vi "探头校准标准值显示.vi"(11 "校准参数":u16(ring) caption="校准参数：" items=["pH", "DO", "浊度", "电导率", "叶绿素a", "藻密度", "ORP", "DO2"]) -> (1 "标液三":sgl, 2 "标液二":sgl, 3 "标液一":sgl)   [LabVIEW 2016, in "斯坦道多参数.lvlib"]
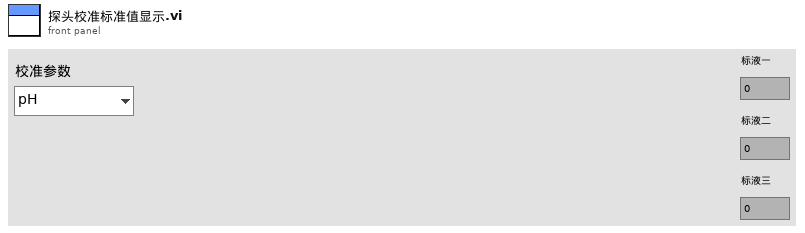
[diagram p1: front panel]
types:
  T1 = cluster{"pH探头选择":u16, "DO探头选择":u16, "电导率探头选择":u16, "浊度探头选择":u16, "叶绿素a探头选择":u16, "蓝绿藻探头选择":u16, "orp探头选择":u16, "COD探头选择":u16, "DO2探头选择":u16}
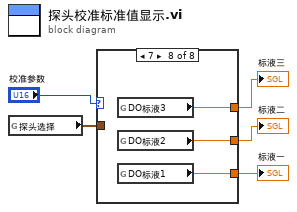
[diagram p0: block diagram]
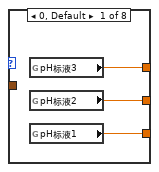
[diagram p2: hidden frame]
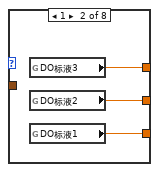
[diagram p3: hidden frame]
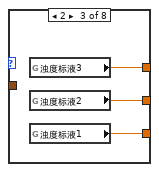
[diagram p4: hidden frame]
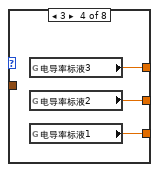
[diagram p5: hidden frame]
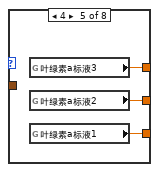
[diagram p6: hidden frame]
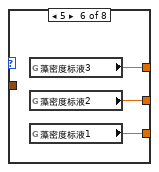
[diagram p7: hidden frame]
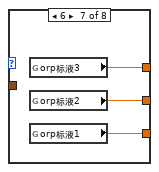
[diagram p8: hidden frame]
diagram:
  n1 = global read "断电保存变量.vi" "探头选择"() -> (w3:T1)
  n2 = case shown="7" "校准参数" {
    tunnel: [w8 w11 w14 w17 w18 w22 w24 w29] -> w5
    tunnel: w3 -> [_ _ _ _ _ _ _ _]
    tunnel: [w7 w10 w13 w16 w19 w21 w25 w28] -> w2
    tunnel: [w6 w9 w12 w15 w20 w23 w26 w27] -> w1
    frame 0, Default {
      n3 = global read "断电保存变量.vi" "pH标液3"() -> (w6:dbl)
      n4 = global read "断电保存变量.vi" "pH标液2"() -> (w7:dbl)
      n5 = global read "断电保存变量.vi" "pH标液1"() -> (w8:dbl)
    }
    frame 1 {
      n6 = global read "断电保存变量.vi" "DO标液3"() -> (w9:dbl)
      n7 = global read "断电保存变量.vi" "DO标液2"() -> (w10:dbl)
      n8 = global read "断电保存变量.vi" "DO标液1"() -> (w11:dbl)
    }
    frame 2 {
      n9 = global read "断电保存变量.vi" "浊度标液3"() -> (w12:dbl)
      n10 = global read "断电保存变量.vi" "浊度标液2"() -> (w13:dbl)
      n11 = global read "断电保存变量.vi" "浊度标液1"() -> (w14:dbl)
    }
    frame 3 {
      n12 = global read "断电保存变量.vi" "电导率标液3"() -> (w15:dbl)
      n13 = global read "断电保存变量.vi" "电导率标液2"() -> (w16:dbl)
      n14 = global read "断电保存变量.vi" "电导率标液1"() -> (w17:dbl)
    }
    frame 4 {
      n15 = global read "断电保存变量.vi" "叶绿素a标液3"() -> (w20:dbl)
      n16 = global read "断电保存变量.vi" "叶绿素a标液2"() -> (w19:dbl)
      n17 = global read "断电保存变量.vi" "叶绿素a标液1"() -> (w18:dbl)
    }
    frame 5 {
      n18 = global read "断电保存变量.vi" "藻密度标液3"() -> (w23:dbl)
      n19 = global read "断电保存变量.vi" "藻密度标液2"() -> (w21:dbl)
      n20 = global read "断电保存变量.vi" "藻密度标液1"() -> (w22:dbl)
    }
    frame 6 {
      n21 = global read "断电保存变量.vi" "orp标液3"() -> (w26:dbl)
      n22 = global read "断电保存变量.vi" "orp标液2"() -> (w25:dbl)
      n23 = global read "断电保存变量.vi" "orp标液1"() -> (w24:dbl)
    }
    frame 7 {
      n24 = global read "断电保存变量.vi" "DO标液3"() -> (w27:dbl)
      n25 = global read "断电保存变量.vi" "DO标液2"() -> (w28:dbl)
      n26 = global read "断电保存变量.vi" "DO标液1"() -> (w29:dbl)
    }
  }
  "标液一" <- w5
  "标液二" <- w2
  "标液三" <- w1
